vi "InitDrivebase.vi"   [LabVIEW 2023]
doc: "This VI initializes devices related directly to the drive subsystem."
uses:
  <vilib>/Rock Robotics/WPI/Solenoid/WPI_SolenoidChannel.ctl
  <vilib>/Rock Robotics/WPI/ThirdParty/Phoenix-LabVIEW/Motor Controller/Controls/CTRE_Phoenix_MotorControl_TalonFXInvertType.ctl
  <vilib>/Rock Robotics/WPI/ThirdParty/Phoenix-LabVIEW/Motor Controller/Controls/CTRE_Phoenix_MotorControl_SupplyCurrentLimitConfiguration.ctl
  <vilib>/Rock Robotics/WPI/ThirdParty/Phoenix-LabVIEW/Motor Controller/Controls/CTRE_Phoenix_MotorControl_NeutralMode.ctl
  <vilib>/Rock Robotics/WPI/ThirdParty/Phoenix-LabVIEW/Motor Controller/Controls/CTRE_Phoenix_MotorControl_FeedbackDevice_TalonFX.ctl
  <vilib>/Rock Robotics/WPI/ThirdParty/Phoenix-LabVIEW/Motor Controller/Controls/CTRE_Phoenix_MotorControl_StatusFrameEnhanced.ctl
  <vilib>/Rock Robotics/WPI/ThirdParty/Phoenix-LabVIEW/Motor Controller/Controls/CTRE_Phoenix_MotorControl_StatorCurrentLimitConfiguration.ctl
  <vilib>/Rock Robotics/WPI/Solenoid/WPI_SolenoidOpenDouble.vi
  GlobalDrivebase.vi
types:
  T1 = typedef "CTRE_Phoenix_MotorControl_StatorCurrentLimitConfiguration.ctl" = cluster{"Enable?":bool, "Current Limit":dbl, "Threshold Current":dbl, "Threshold Time":dbl}
  T2 = typedef "CTRE_Phoenix_MotorControl_StatusFrameEnhanced.ctl" = u16
  T3 = typedef "WPI_SolenoidChannel.ctl" = enum8{"Solenoid 0", "Solenoid 1", "Solenoid 2", "Solenoid 3", "Solenoid 4", "Solenoid 5", "Solenoid 6", "Solenoid 7", "Solenoid 8", "Solenoid 9", "Solenoid 10", "Solenoid 11", "Solenoid 12", "Solenoid 13", "Solenoid 14", "Solenoid 15", "Invalid"}
  T4 = typedef "CTRE_Phoenix_MotorControl_TalonFXInvertType.ctl" = enum16{"Counter-Clockwise", "Clockwise"}
  T5 = typedef "CTRE_Phoenix_MotorControl_FeedbackDevice_TalonFX.ctl" = i8
  T6 = typedef "CTRE_Phoenix_MotorControl_SupplyCurrentLimitConfiguration.ctl" = cluster{"Enable?":bool, "Current Limit":dbl, "Threshold Current":dbl, "Threshold Time":dbl}
  T7 = typedef "CTRE_Phoenix_MotorControl_NeutralMode.ctl" = enum8{"EEPROMSetting", "Override to Coast", "Override to Brake"}
  T8 = typedef "CTRE_PigeonIMU_DeviceRef.ctl" = cluster{"DeviceStatus":errorcluster, "Device Number":u8, "Type":T9, "Device ID":u32, "Handle":u64, "UsageFrame":u32, "Library Path":path}
  T9 = typedef "CTRE_PigeonIMU_ConnectionType.ctl" = u32
  T10 = typedef "WPI_MotorControlDeviceRef.ctl" = cluster{"DeviceStatus":errorcluster, "Type":T11, "PWM":cluster{"PWM Channel":T12, "DeadBand":T13}, "CAN":cluster{"Device Number":u8, "SetOutput VI Ref":variant, "GetOutput VI Ref":variant, "Enable VI Ref":variant, "Disable VI Ref":variant, "Data":variant}, "Invert":bool, "DIO PWM":cluster{"PWM \"Enable\" Channel":T12, "DIOChannel":T14, "PWM Rate":dbl}}
  T11 = typedef "WPI_MotorControlType.ctl" = enum16{"PWM", "CAN", "DIO PWM"}
  T12 = typedef "FPGA_DIOPWMChannel.ctl" = enum8{"PWM 0", "PWM 1", "PWM 2", "PWM 3", "PWM 4", "PWM 5", "PWM 6", "PWM 7", "PWM 8", "PWM 9", "PWM MXP 0", "PWM MXP 1", "PWM MXP 2", "PWM MXP 3", "PWM MXP 4", "PWM MXP 5", "PWM MXP 6", "PWM MXP 7", "PWM MXP 8", "PWM MXP 9", "Invalid"}
  T13 = typedef "WPI_PWMDeadband.ctl" = cluster{"Name":string, "maxPositivePwm":i32, "minPositivePwm":i32, "centerPwm":i32, "maxNegativePwm":i32, "minNegativePwm":i32, "angularRange":u16}
  T14 = typedef "FPGA_DIOChannel.ctl" = enum8{"DIO 0", "DIO 1", "DIO 2", "DIO 3", "DIO 4", "DIO 5", "DIO 6", "DIO 7", "DIO 8", "DIO 9", "DIO MXP 0", "DIO MXP 1", "DIO MXP 2", "DIO MXP 3", "DIO MXP 4", "DIO MXP 5", "DIO MXP 6", "DIO MXP 7", "DIO MXP 8", "DIO MXP 9", "DIO MXP 10", "DIO MXP 11", "DIO MXP 12", "DIO MXP 13", "DIO MXP 14", "DIO MXP 15", "SPI Port CS1", "SPI Port CS2", "SPI Port CS3", "SPI Port MISO", "SPI Port MOSI", "Invalid"}
  T15 = typedef "WPI_SolenoidDevRef.ctl" = cluster{"DevStatus":errorcluster, "Pneumatics Control Module":u8, "Forward Solenoid Channel":T3, "Reverse Solenoid Channel":T3}
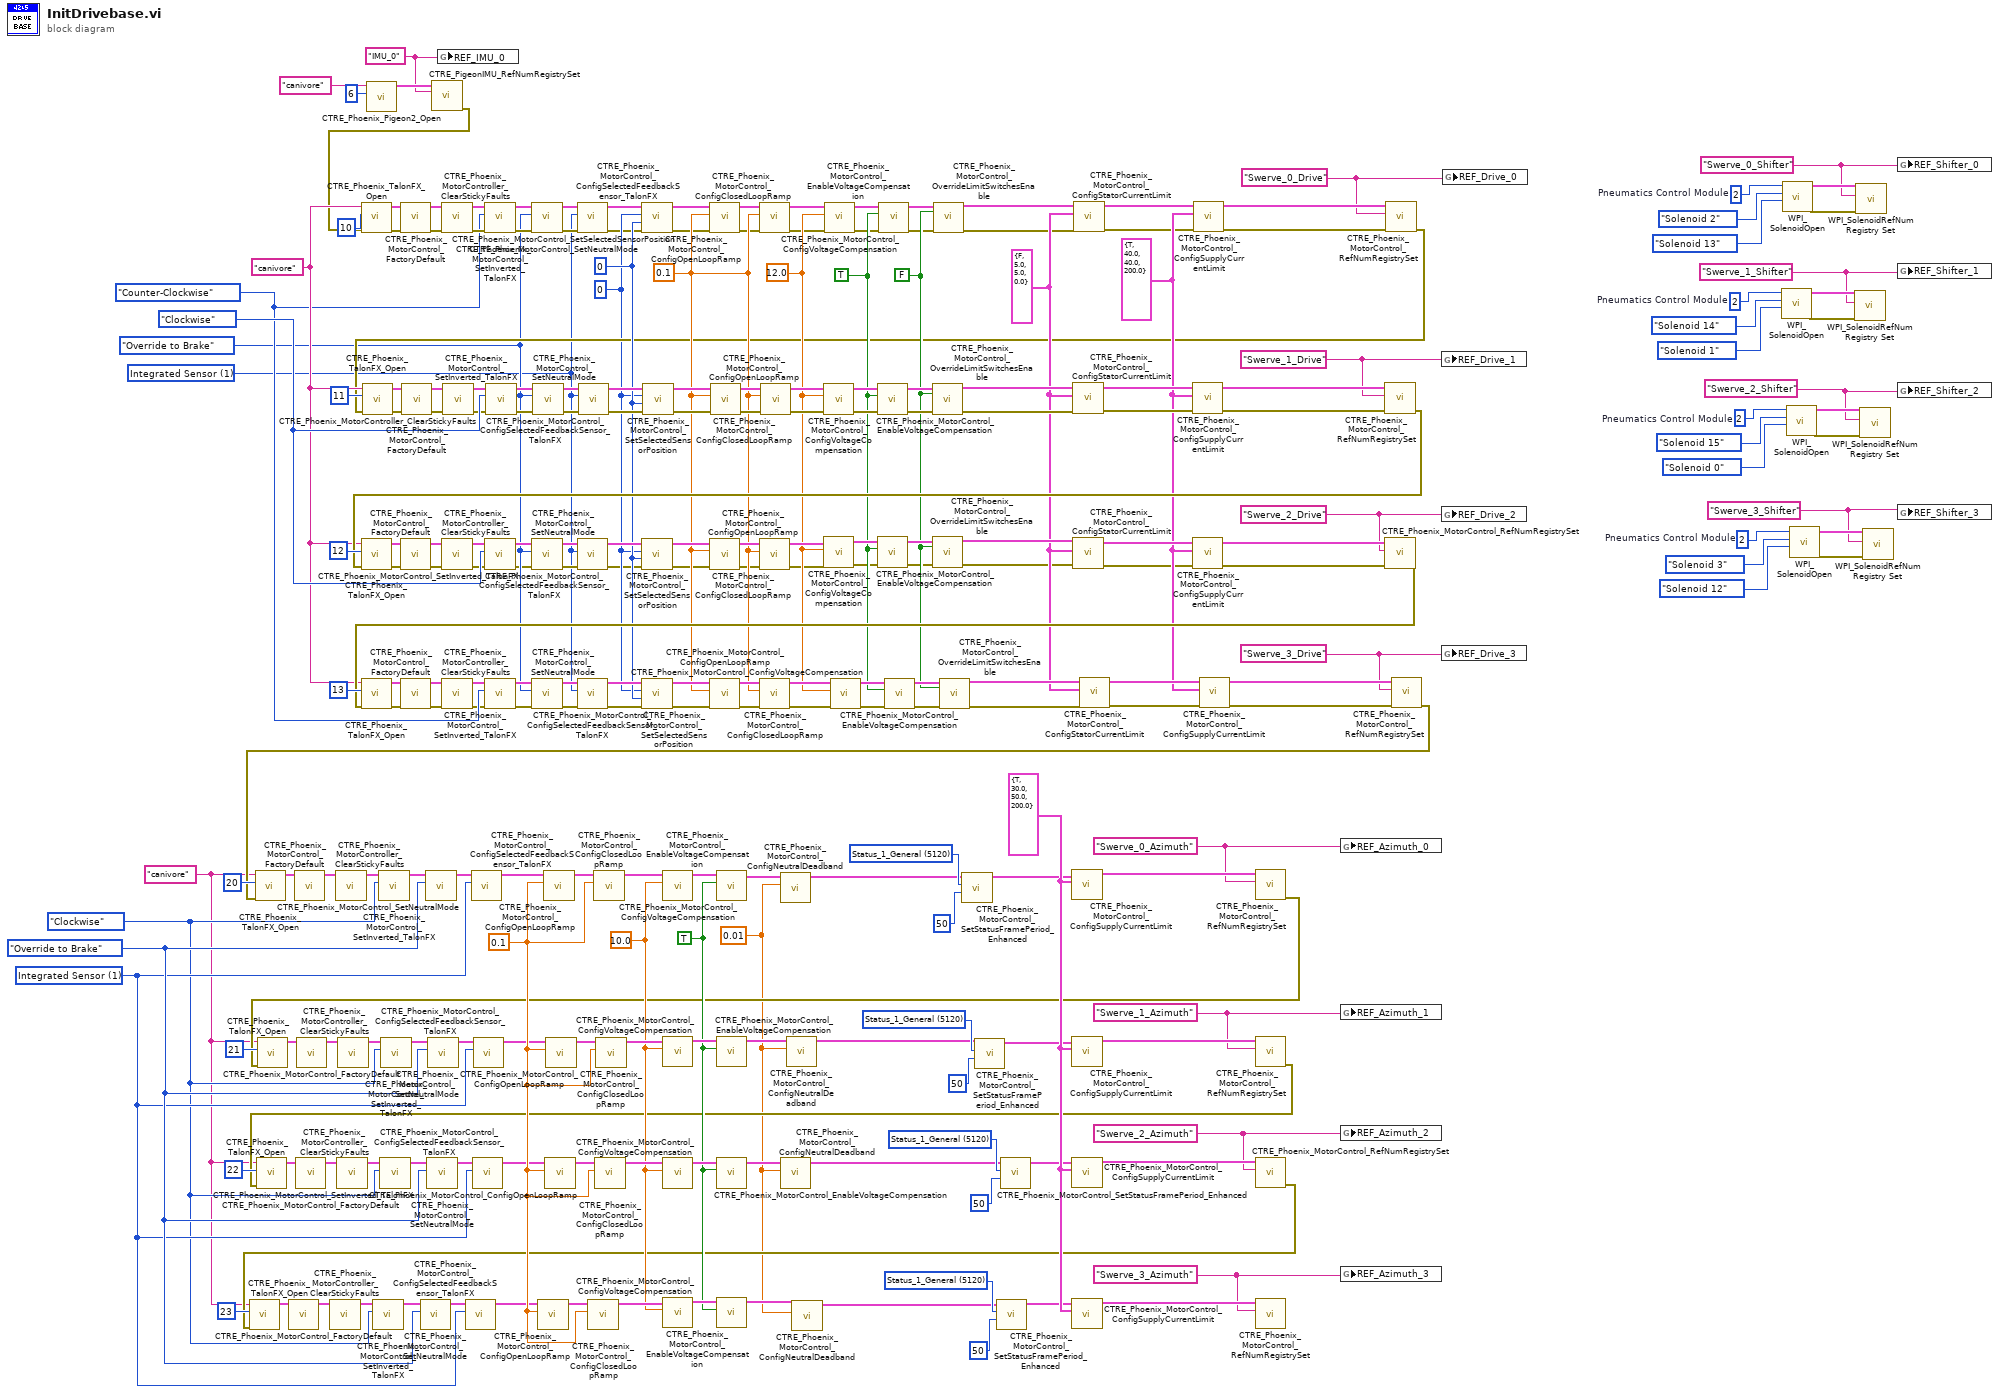
[diagram p0: block diagram]
diagram:
  w35 = "Swerve_0_Drive" ("refnum name")
  w64 = 0 ("New Sensor Position")
  w88 = "canivore" ("CAN Bus")
  w66 = "canivore" ("CAN Bus")
  w89 = "IMU_0" ("refnum name")
  w106 = 0.01 ("Percent Deadband")
  w73 = T1 {"Enable?"=FALSE, "Current Limit"=5.0, "Threshold Current"=5.0, "Threshold Time"=0.0} ("Stator Current Limit Configuration")
  w122 = T2 5120 items=["Status_1_General"=5120, "Status_2_Feedback0"=5184, "Status_3_Quadrature"=5248, "Status_4_AinTempVbat"=5312, "Status_6_Misc"=5440, "Status_7_CommStatus"=5504, "Status_8_PulseWidth"=5568, "Status_9_MotProfBuffer"=5632, "Status_10_MotionMagic"=5696, "Status_11_UartGadgeteer"=5760, "Status_12_Feedback1"=5824, "Status_13_Base_PIDF0"=5888, "Status_14_Turn_PIDF1"=5952, "Status_15_FirmwareApiStatus"=6016, "Status_Brushless_Current"=4672] ("Status Frame")
  w125 = T2 5120 items=["Status_1_General"=5120, "Status_2_Feedback0"=5184, "Status_3_Quadrature"=5248, "Status_4_AinTempVbat"=5312, "Status_6_Misc"=5440, "Status_7_CommStatus"=5504, "Status_8_PulseWidth"=5568, "Status_9_MotProfBuffer"=5632, "Status_10_MotionMagic"=5696, "Status_11_UartGadgeteer"=5760, "Status_12_Feedback1"=5824, "Status_13_Base_PIDF0"=5888, "Status_14_Turn_PIDF1"=5952, "Status_15_FirmwareApiStatus"=6016, "Status_Brushless_Current"=4672] ("Status Frame")
  w128 = T2 5120 items=["Status_1_General"=5120, "Status_2_Feedback0"=5184, "Status_3_Quadrature"=5248, "Status_4_AinTempVbat"=5312, "Status_6_Misc"=5440, "Status_7_CommStatus"=5504, "Status_8_PulseWidth"=5568, "Status_9_MotProfBuffer"=5632, "Status_10_MotionMagic"=5696, "Status_11_UartGadgeteer"=5760, "Status_12_Feedback1"=5824, "Status_13_Base_PIDF0"=5888, "Status_14_Turn_PIDF1"=5952, "Status_15_FirmwareApiStatus"=6016, "Status_Brushless_Current"=4672] ("Status Frame")
  w130 = T2 5120 items=["Status_1_General"=5120, "Status_2_Feedback0"=5184, "Status_3_Quadrature"=5248, "Status_4_AinTempVbat"=5312, "Status_6_Misc"=5440, "Status_7_CommStatus"=5504, "Status_8_PulseWidth"=5568, "Status_9_MotProfBuffer"=5632, "Status_10_MotionMagic"=5696, "Status_11_UartGadgeteer"=5760, "Status_12_Feedback1"=5824, "Status_13_Base_PIDF0"=5888, "Status_14_Turn_PIDF1"=5952, "Status_15_FirmwareApiStatus"=6016, "Status_Brushless_Current"=4672] ("Status Frame")
  w72 = FALSE ("Override Limit Switch Enable?")
  w100 = "Swerve_0_Shifter" ("refnum name")
  w148 = u8 2  # Pneumatics Control Module
  w99 = "Swerve_1_Shifter" ("refnum name")
  w153 = u8 2  # Pneumatics Control Module
  w98 = "Swerve_2_Shifter" ("refnum name")
  w158 = u8 2  # Pneumatics Control Module
  w32 = CTRE_Phoenix_MotorControl_TalonFXInvertType."Counter-Clockwise" ("Invert Type")
  w160 = TRUE ("Enable Voltage Compensation?")
  w161 = 10.0 ("Saturation Voltage")
  w71 = TRUE ("Enable Voltage Compensation?")
  w70 = 12.0 ("Saturation Voltage")
  w176 = T5 1 items=["Integrated Sensor"=1, "Sensor Sum (S0 + S1)"=9, "Sensor Difference (D0 - D1)"=10, "Remote Source 0"=11, "Remote Source 1"=12, "None"=14, "Software Emulated"=15] ("Talon FX Feedback Device")
  w179 = T6 {"Enable?"=TRUE, "Current Limit"=30.0, "Threshold Current"=50.0, "Threshold Time"=200.0} ("Supply Current Limit Configuration")
  w177 = 0.1 ("secondsFromNeutralToFull")
  w178 = CTRE_Phoenix_MotorControl_NeutralMode."Override to Brake" ("Motor Control Neutral Mode")
  w143 = CTRE_Phoenix_MotorControl_TalonFXInvertType."Clockwise" ("Invert Type")
  w93 = "Swerve_0_Azimuth" ("refnum name")
  w92 = "Swerve_1_Azimuth" ("refnum name")
  w91 = "Swerve_2_Azimuth" ("refnum name")
  w90 = "Swerve_3_Azimuth" ("refnum name")
  w1 = T5 1 items=["Integrated Sensor"=1, "Sensor Sum (S0 + S1)"=9, "Sensor Difference (D0 - D1)"=10, "Remote Source 0"=11, "Remote Source 1"=12, "None"=14, "Software Emulated"=15] ("Talon FX Feedback Device")
  w69 = T6 {"Enable?"=TRUE, "Current Limit"=40.0, "Threshold Current"=40.0, "Threshold Time"=200.0} ("Supply Current Limit Configuration")
  w68 = 0.1 ("secondsFromNeutralToFull")
  w67 = u32 0 ("pidLoopIdx")
  w31 = CTRE_Phoenix_MotorControl_NeutralMode."Override to Brake" ("Motor Control Neutral Mode")
  w159 = CTRE_Phoenix_MotorControl_TalonFXInvertType."Clockwise" ("Invert Type")
  w96 = "Swerve_1_Drive" ("refnum name")
  w95 = "Swerve_2_Drive" ("refnum name")
  w94 = "Swerve_3_Drive" ("refnum name")
  w97 = "Swerve_3_Shifter" ("refnum name")
  w246 = u8 2  # Pneumatics Control Module
  n1 = call <vilib>:"CTRE_Phoenix_Pigeon2_Open.vi"("Device Number"=u8 6, "canbus"="canivore") -> ("PigeonIMUDevRef"=w104:T8)  [unwired: 8 in, 1 out]
  n2 = call <vilib>:"CTRE_PigeonIMU_RefNumRegistrySet.vi"("refnum name"=w89, "PigeonIMUDevRef"=w104) -> ("error out"=w33:errorcluster)  [unwired: 8 in, 1 out]
  n3 = call <vilib>:"CTRE_Phoenix_TalonFX_Open.vi"("error in"=w33, "Device Number"=u8 10 ("Drive 4L"), "CAN Bus"=w66) -> ("error out"=w50:errorcluster, "PhoenixMotorControlDevRef"=w39:T10)  [unwired: 7 in]
  n4 = call <vilib>:"CTRE_Phoenix_MotorControl_FactoryDefault.vi"("error in"=w50, "PhoenixMotorControlDevRef"=w39) -> ("error out"=w51:errorcluster, "PhoenixMotorControlDevRef"=w41:T10)  [unwired: 8 in]
  n5 = global write "GlobalDrivebase.vi" "REF_IMU_0"(w89) -> ()
  n6 = call <vilib>:"CTRE_Phoenix_MotorController_ClearStickyFaults.vi"("error in"=w51, "PhoenixMotorControlDevRef"=w41) -> ("error out"=w52:errorcluster, "PhoenixMotorControlDevRef"=w42:T10)  [unwired: 8 in]
  n7 = call <vilib>:"CTRE_Phoenix_MotorControl_SetInverted_TalonFX.vi"("error in (no error)"=w52, "Invert Type"=w32, "PhoenixMotorControlDevRef"=w42) -> ("error out"=w53:errorcluster, "PhoenixMotorControlDevRef"=w36:T10)  [unwired: 7 in]
  n8 = call <vilib>:"CTRE_Phoenix_MotorControl_SetNeutralMode.vi"("error in (no error)"=w53, "Motor Control Neutral Mode"=w31, "PhoenixMotorControlDevRef"=w36) -> ("error out"=w54:errorcluster, "PhoenixMotorControlDevRef"=w43:T10)  [unwired: 7 in]
  n9 = call <vilib>:"CTRE_Phoenix_MotorControl_ConfigSelectedFeedbackSensor_TalonFX.vi"("error in (no error)"=w54, "Talon FX Feedback Device"=w1, "PhoenixMotorControlDevRef"=w43) -> ("error out"=w55:errorcluster, "PhoenixMotorControlDevRef"=w44:T10)  [unwired: 7 in]
  n10 = call <vilib>:"CTRE_Phoenix_MotorControl_SetSelectedSensorPosition.vi"("error in (no error)"=w55, "pidLoopIdx"=w67, "New Sensor Position"=w64, "PhoenixMotorControlDevRef"=w44) -> ("error out"=w56:errorcluster, "PhoenixMotorControlDevRef"=w37:T10)  [unwired: 6 in]
  n11 = call <vilib>:"CTRE_Phoenix_MotorControl_ConfigOpenLoopRamp.vi"("error in (no error)"=w56, "secondsFromNeutralToFull"=w68, "PhoenixMotorControlDevRef"=w37) -> ("error out"=w57:errorcluster, "PhoenixMotorControlDevRef"=w40:T10)  [unwired: 7 in]
  n12 = call <vilib>:"CTRE_Phoenix_MotorControl_ConfigClosedLoopRamp.vi"("error in (no error)"=w57, "secondsFromNeutralToFull"=w68, "PhoenixMotorControlDevRef"=w40) -> ("error out"=w58:errorcluster, "PhoenixMotorControlDevRef"=w46:T10)  [unwired: 7 in]
  n13 = call <vilib>:"CTRE_Phoenix_MotorControl_ConfigVoltageCompensation.vi"("error in (no error)"=w58, "Saturation Voltage"=w70, "PhoenixMotorControlDevRef"=w46) -> ("error out"=w59:errorcluster, "PhoenixMotorControlDevRef"=w45:T10)  [unwired: 7 in]
  n14 = call <vilib>:"CTRE_Phoenix_MotorControl_EnableVoltageCompensation.vi"("error in (no error)"=w59, "Enable Voltage Compensation?"=w71, "PhoenixMotorControlDevRef"=w45) -> ("error out"=w60:errorcluster, "PhoenixMotorControlDevRef"=w47:T10)  [unwired: 7 in]
  n15 = call <vilib>:"CTRE_Phoenix_MotorControl_OverrideLimitSwitchesEnable.vi"("PhoenixMotorControlDevRef"=w47, "Override Limit Switch Enable?"=w72, "error in (no error)"=w60) -> ("PhoenixMotorControlDevRef"=w49:T10, "error out"=w61:errorcluster)  [unwired: 11 in]
  n16 = call <vilib>:"CTRE_Phoenix_MotorControl_ConfigStatorCurrentLimit.vi"("error in (no error)"=w61, "Stator Current Limit Configuration"=w73, "PhoenixMotorControlDevRef"=w49) -> ("error out"=w62:errorcluster, "PhoenixMotorControlDevRef"=w48:T10)  [unwired: 7 in]
  n17 = call <vilib>:"CTRE_Phoenix_MotorControl_ConfigSupplyCurrentLimit.vi"("error in (no error)"=w62, "Supply Current Limit Configuration"=w69, "PhoenixMotorControlDevRef"=w48) -> ("error out"=w63:errorcluster, "PhoenixMotorControlDevRef"=w38:T10)  [unwired: 7 in]
  n18 = global write "GlobalDrivebase.vi" "REF_Azimuth_0"(w93) -> ()
  n19 = global write "GlobalDrivebase.vi" "REF_Azimuth_1"(w92) -> ()
  n20 = global write "GlobalDrivebase.vi" "REF_Azimuth_2"(w91) -> ()
  n21 = global write "GlobalDrivebase.vi" "REF_Azimuth_3"(w90) -> ()
  n22 = call <vilib>:"CTRE_Phoenix_MotorControl_RefNumRegistrySet.vi"("error in (no error)"=w63, "refnum name"=w35, "PhoenixMotorControlDevRef"=w38) -> ("error out"=w65:errorcluster)  [unwired: 7 in, 1 out]
  n23 = call <vilib>:"CTRE_Phoenix_TalonFX_Open.vi"("error in"=w65, "Device Number"=u8 11 ("Drive 4L"), "CAN Bus"=w66) -> ("error out"=w86:errorcluster, "PhoenixMotorControlDevRef"=w217:T10)  [unwired: 7 in]
  n24 = call <vilib>:"CTRE_Phoenix_MotorControl_FactoryDefault.vi"("error in"=w86, "PhoenixMotorControlDevRef"=w217) -> ("error out"=w85:errorcluster, "PhoenixMotorControlDevRef"=w215:T10)  [unwired: 8 in]
  n25 = call <vilib>:"CTRE_Phoenix_MotorController_ClearStickyFaults.vi"("error in"=w85, "PhoenixMotorControlDevRef"=w215) -> ("error out"=w84:errorcluster, "PhoenixMotorControlDevRef"=w214:T10)  [unwired: 8 in]
  n26 = call <vilib>:"CTRE_Phoenix_MotorControl_SetInverted_TalonFX.vi"("error in (no error)"=w84, "Invert Type"=w159, "PhoenixMotorControlDevRef"=w214) -> ("error out"=w83:errorcluster, "PhoenixMotorControlDevRef"=w221:T10)  [unwired: 7 in]
  n27 = call <vilib>:"CTRE_Phoenix_MotorControl_SetNeutralMode.vi"("error in (no error)"=w83, "Motor Control Neutral Mode"=w31, "PhoenixMotorControlDevRef"=w221) -> ("error out"=w82:errorcluster, "PhoenixMotorControlDevRef"=w213:T10)  [unwired: 7 in]
  n28 = call <vilib>:"CTRE_Phoenix_MotorControl_ConfigSelectedFeedbackSensor_TalonFX.vi"("error in (no error)"=w82, "Talon FX Feedback Device"=w1, "PhoenixMotorControlDevRef"=w213) -> ("error out"=w81:errorcluster, "PhoenixMotorControlDevRef"=w212:T10)  [unwired: 7 in]
  n29 = call <vilib>:"CTRE_Phoenix_MotorControl_SetSelectedSensorPosition.vi"("error in (no error)"=w81, "pidLoopIdx"=w67, "New Sensor Position"=w64, "PhoenixMotorControlDevRef"=w212) -> ("error out"=w80:errorcluster, "PhoenixMotorControlDevRef"=w220:T10)  [unwired: 6 in]
  n30 = call <vilib>:"CTRE_Phoenix_MotorControl_ConfigOpenLoopRamp.vi"("error in (no error)"=w80, "secondsFromNeutralToFull"=w68, "PhoenixMotorControlDevRef"=w220) -> ("error out"=w79:errorcluster, "PhoenixMotorControlDevRef"=w216:T10)  [unwired: 7 in]
  n31 = call <vilib>:"CTRE_Phoenix_MotorControl_ConfigClosedLoopRamp.vi"("error in (no error)"=w79, "secondsFromNeutralToFull"=w68, "PhoenixMotorControlDevRef"=w216) -> ("error out"=w78:errorcluster, "PhoenixMotorControlDevRef"=w168:T10)  [unwired: 7 in]
  n32 = call <vilib>:"CTRE_Phoenix_MotorControl_ConfigVoltageCompensation.vi"("error in (no error)"=w78, "Saturation Voltage"=w70, "PhoenixMotorControlDevRef"=w168) -> ("error out"=w77:errorcluster, "PhoenixMotorControlDevRef"=w175:T10)  [unwired: 7 in]
  n33 = call <vilib>:"CTRE_Phoenix_MotorControl_EnableVoltageCompensation.vi"("error in (no error)"=w77, "Enable Voltage Compensation?"=w71, "PhoenixMotorControlDevRef"=w175) -> ("error out"=w76:errorcluster, "PhoenixMotorControlDevRef"=w142:T10)  [unwired: 7 in]
  n34 = call <vilib>:"CTRE_Phoenix_MotorControl_OverrideLimitSwitchesEnable.vi"("PhoenixMotorControlDevRef"=w142, "Override Limit Switch Enable?"=w72, "error in (no error)"=w76) -> ("PhoenixMotorControlDevRef"=w117:T10, "error out"=w75:errorcluster)  [unwired: 11 in]
  n35 = call <vilib>:"CTRE_Phoenix_MotorControl_ConfigStatorCurrentLimit.vi"("error in (no error)"=w75, "Stator Current Limit Configuration"=w73, "PhoenixMotorControlDevRef"=w117) -> ("error out"=w74:errorcluster, "PhoenixMotorControlDevRef"=w120:T10)  [unwired: 7 in]
  n36 = call <vilib>:"CTRE_Phoenix_MotorControl_ConfigSupplyCurrentLimit.vi"("error in (no error)"=w74, "Supply Current Limit Configuration"=w69, "PhoenixMotorControlDevRef"=w120) -> ("error out"=w30:errorcluster, "PhoenixMotorControlDevRef"=w219:T10)  [unwired: 7 in]
  n37 = call <vilib>:"CTRE_Phoenix_MotorControl_RefNumRegistrySet.vi"("error in (no error)"=w30, "refnum name"=w96, "PhoenixMotorControlDevRef"=w219) -> ("error out"=w103:errorcluster)  [unwired: 7 in, 1 out]
  n38 = call <vilib>:"CTRE_Phoenix_TalonFX_Open.vi"("error in"=w103, "Device Number"=u8 12 ("Drive 4L"), "CAN Bus"=w66) -> ("error out"=w29:errorcluster, "PhoenixMotorControlDevRef"=w227:T10)  [unwired: 7 in]
  n39 = call <vilib>:"CTRE_Phoenix_MotorControl_FactoryDefault.vi"("error in"=w29, "PhoenixMotorControlDevRef"=w227) -> ("error out"=w28:errorcluster, "PhoenixMotorControlDevRef"=w225:T10)  [unwired: 8 in]
  n40 = call <vilib>:"CTRE_Phoenix_MotorController_ClearStickyFaults.vi"("error in"=w28, "PhoenixMotorControlDevRef"=w225) -> ("error out"=w27:errorcluster, "PhoenixMotorControlDevRef"=w224:T10)  [unwired: 8 in]
  n41 = call <vilib>:"CTRE_Phoenix_MotorControl_SetInverted_TalonFX.vi"("error in (no error)"=w27, "Invert Type"=w159, "PhoenixMotorControlDevRef"=w224) -> ("error out"=w26:errorcluster, "PhoenixMotorControlDevRef"=w231:T10)  [unwired: 7 in]
  n42 = call <vilib>:"CTRE_Phoenix_MotorControl_SetNeutralMode.vi"("error in (no error)"=w26, "Motor Control Neutral Mode"=w31, "PhoenixMotorControlDevRef"=w231) -> ("error out"=w25:errorcluster, "PhoenixMotorControlDevRef"=w223:T10)  [unwired: 7 in]
  n43 = call <vilib>:"CTRE_Phoenix_MotorControl_ConfigSelectedFeedbackSensor_TalonFX.vi"("error in (no error)"=w25, "Talon FX Feedback Device"=w1, "PhoenixMotorControlDevRef"=w223) -> ("error out"=w24:errorcluster, "PhoenixMotorControlDevRef"=w222:T10)  [unwired: 7 in]
  n44 = call <vilib>:"CTRE_Phoenix_MotorControl_SetSelectedSensorPosition.vi"("error in (no error)"=w24, "pidLoopIdx"=w67, "New Sensor Position"=w64, "PhoenixMotorControlDevRef"=w222) -> ("error out"=w23:errorcluster, "PhoenixMotorControlDevRef"=w230:T10)  [unwired: 6 in]
  n45 = call <vilib>:"CTRE_Phoenix_MotorControl_ConfigOpenLoopRamp.vi"("error in (no error)"=w23, "secondsFromNeutralToFull"=w68, "PhoenixMotorControlDevRef"=w230) -> ("error out"=w22:errorcluster, "PhoenixMotorControlDevRef"=w226:T10)  [unwired: 7 in]
  n46 = call <vilib>:"CTRE_Phoenix_MotorControl_ConfigClosedLoopRamp.vi"("error in (no error)"=w22, "secondsFromNeutralToFull"=w68, "PhoenixMotorControlDevRef"=w226) -> ("error out"=w21:errorcluster, "PhoenixMotorControlDevRef"=w167:T10)  [unwired: 7 in]
  n47 = call <vilib>:"CTRE_Phoenix_MotorControl_ConfigVoltageCompensation.vi"("error in (no error)"=w21, "Saturation Voltage"=w70, "PhoenixMotorControlDevRef"=w167) -> ("error out"=w20:errorcluster, "PhoenixMotorControlDevRef"=w174:T10)  [unwired: 7 in]
  n48 = call <vilib>:"CTRE_Phoenix_MotorControl_EnableVoltageCompensation.vi"("error in (no error)"=w20, "Enable Voltage Compensation?"=w71, "PhoenixMotorControlDevRef"=w174) -> ("error out"=w19:errorcluster, "PhoenixMotorControlDevRef"=w141:T10)  [unwired: 7 in]
  n49 = call <vilib>:"CTRE_Phoenix_MotorControl_OverrideLimitSwitchesEnable.vi"("PhoenixMotorControlDevRef"=w141, "Override Limit Switch Enable?"=w72, "error in (no error)"=w19) -> ("PhoenixMotorControlDevRef"=w116:T10, "error out"=w18:errorcluster)  [unwired: 11 in]
  n50 = call <vilib>:"CTRE_Phoenix_MotorControl_ConfigStatorCurrentLimit.vi"("error in (no error)"=w18, "Stator Current Limit Configuration"=w73, "PhoenixMotorControlDevRef"=w116) -> ("error out"=w17:errorcluster, "PhoenixMotorControlDevRef"=w119:T10)  [unwired: 7 in]
  n51 = call <vilib>:"CTRE_Phoenix_MotorControl_ConfigSupplyCurrentLimit.vi"("error in (no error)"=w17, "Supply Current Limit Configuration"=w69, "PhoenixMotorControlDevRef"=w119) -> ("error out"=w16:errorcluster, "PhoenixMotorControlDevRef"=w229:T10)  [unwired: 7 in]
  n52 = call <vilib>:"CTRE_Phoenix_MotorControl_RefNumRegistrySet.vi"("error in (no error)"=w16, "refnum name"=w95, "PhoenixMotorControlDevRef"=w229) -> ("error out"=w102:errorcluster)  [unwired: 7 in, 1 out]
  n53 = call <vilib>:"CTRE_Phoenix_TalonFX_Open.vi"("error in"=w102, "Device Number"=u8 13 ("Drive 4L"), "CAN Bus"=w66) -> ("error out"=w15:errorcluster, "PhoenixMotorControlDevRef"=w237:T10)  [unwired: 7 in]
  n54 = call <vilib>:"CTRE_Phoenix_MotorControl_FactoryDefault.vi"("error in"=w15, "PhoenixMotorControlDevRef"=w237) -> ("error out"=w14:errorcluster, "PhoenixMotorControlDevRef"=w235:T10)  [unwired: 8 in]
  n55 = call <vilib>:"CTRE_Phoenix_MotorController_ClearStickyFaults.vi"("error in"=w14, "PhoenixMotorControlDevRef"=w235) -> ("error out"=w13:errorcluster, "PhoenixMotorControlDevRef"=w234:T10)  [unwired: 8 in]
  n56 = call <vilib>:"CTRE_Phoenix_MotorControl_SetInverted_TalonFX.vi"("error in (no error)"=w13, "Invert Type"=w32, "PhoenixMotorControlDevRef"=w234) -> ("error out"=w12:errorcluster, "PhoenixMotorControlDevRef"=w241:T10)  [unwired: 7 in]
  n57 = call <vilib>:"CTRE_Phoenix_MotorControl_SetNeutralMode.vi"("error in (no error)"=w12, "Motor Control Neutral Mode"=w31, "PhoenixMotorControlDevRef"=w241) -> ("error out"=w11:errorcluster, "PhoenixMotorControlDevRef"=w233:T10)  [unwired: 7 in]
  n58 = call <vilib>:"CTRE_Phoenix_MotorControl_ConfigSelectedFeedbackSensor_TalonFX.vi"("error in (no error)"=w11, "Talon FX Feedback Device"=w1, "PhoenixMotorControlDevRef"=w233) -> ("error out"=w10:errorcluster, "PhoenixMotorControlDevRef"=w232:T10)  [unwired: 7 in]
  n59 = call <vilib>:"CTRE_Phoenix_MotorControl_SetSelectedSensorPosition.vi"("error in (no error)"=w10, "pidLoopIdx"=w67, "New Sensor Position"=w64, "PhoenixMotorControlDevRef"=w232) -> ("error out"=w9:errorcluster, "PhoenixMotorControlDevRef"=w240:T10)  [unwired: 6 in]
  n60 = call <vilib>:"CTRE_Phoenix_MotorControl_ConfigOpenLoopRamp.vi"("error in (no error)"=w9, "secondsFromNeutralToFull"=w68, "PhoenixMotorControlDevRef"=w240) -> ("error out"=w8:errorcluster, "PhoenixMotorControlDevRef"=w236:T10)  [unwired: 7 in]
  n61 = call <vilib>:"CTRE_Phoenix_MotorControl_ConfigClosedLoopRamp.vi"("error in (no error)"=w8, "secondsFromNeutralToFull"=w68, "PhoenixMotorControlDevRef"=w236) -> ("error out"=w7:errorcluster, "PhoenixMotorControlDevRef"=w166:T10)  [unwired: 7 in]
  n62 = call <vilib>:"CTRE_Phoenix_MotorControl_ConfigVoltageCompensation.vi"("error in (no error)"=w7, "Saturation Voltage"=w70, "PhoenixMotorControlDevRef"=w166) -> ("error out"=w6:errorcluster, "PhoenixMotorControlDevRef"=w173:T10)  [unwired: 7 in]
  n63 = call <vilib>:"CTRE_Phoenix_MotorControl_EnableVoltageCompensation.vi"("error in (no error)"=w6, "Enable Voltage Compensation?"=w71, "PhoenixMotorControlDevRef"=w173) -> ("error out"=w5:errorcluster, "PhoenixMotorControlDevRef"=w140:T10)  [unwired: 7 in]
  n64 = call <vilib>:"CTRE_Phoenix_MotorControl_OverrideLimitSwitchesEnable.vi"("PhoenixMotorControlDevRef"=w140, "Override Limit Switch Enable?"=w72, "error in (no error)"=w5) -> ("PhoenixMotorControlDevRef"=w115:T10, "error out"=w4:errorcluster)  [unwired: 11 in]
  n65 = call <vilib>:"CTRE_Phoenix_MotorControl_ConfigStatorCurrentLimit.vi"("error in (no error)"=w4, "Stator Current Limit Configuration"=w73, "PhoenixMotorControlDevRef"=w115) -> ("error out"=w3:errorcluster, "PhoenixMotorControlDevRef"=w118:T10)  [unwired: 7 in]
  n66 = call <vilib>:"CTRE_Phoenix_MotorControl_ConfigSupplyCurrentLimit.vi"("error in (no error)"=w3, "Supply Current Limit Configuration"=w69, "PhoenixMotorControlDevRef"=w118) -> ("error out"=w2:errorcluster, "PhoenixMotorControlDevRef"=w239:T10)  [unwired: 7 in]
  n67 = call <vilib>:"CTRE_Phoenix_MotorControl_RefNumRegistrySet.vi"("error in (no error)"=w2, "refnum name"=w94, "PhoenixMotorControlDevRef"=w239) -> ("error out"=w101:errorcluster)  [unwired: 7 in, 1 out]
  n68 = call <vilib>:"CTRE_Phoenix_TalonFX_Open.vi"("error in"=w101, "Device Number"=u8 20 ("Drive 4L"), "CAN Bus"=w88) -> ("PhoenixMotorControlDevRef"=w184:T10)  [unwired: 7 in, 1 out]
  n69 = call <vilib>:"CTRE_Phoenix_MotorControl_FactoryDefault.vi"("PhoenixMotorControlDevRef"=w184) -> ("PhoenixMotorControlDevRef"=w182:T10)  [unwired: 9 in, 1 out]
  n70 = call <vilib>:"CTRE_Phoenix_MotorController_ClearStickyFaults.vi"("PhoenixMotorControlDevRef"=w182) -> ("PhoenixMotorControlDevRef"=w181:T10)  [unwired: 9 in, 1 out]
  n71 = call <vilib>:"CTRE_Phoenix_MotorControl_SetInverted_TalonFX.vi"("Invert Type"=w143, "PhoenixMotorControlDevRef"=w181) -> ("PhoenixMotorControlDevRef"=w187:T10)  [unwired: 8 in, 1 out]
  n72 = call <vilib>:"CTRE_Phoenix_MotorControl_SetNeutralMode.vi"("Motor Control Neutral Mode"=w178, "PhoenixMotorControlDevRef"=w187) -> ("PhoenixMotorControlDevRef"=w180:T10)  [unwired: 8 in, 1 out]
  n73 = call <vilib>:"CTRE_Phoenix_MotorControl_ConfigSelectedFeedbackSensor_TalonFX.vi"("Talon FX Feedback Device"=w176, "PhoenixMotorControlDevRef"=w180) -> ("PhoenixMotorControlDevRef"=w136:T10)  [unwired: 8 in, 1 out]
  n74 = call <vilib>:"CTRE_Phoenix_MotorControl_ConfigOpenLoopRamp.vi"("secondsFromNeutralToFull"=w177, "PhoenixMotorControlDevRef"=w136) -> ("PhoenixMotorControlDevRef"=w183:T10)  [unwired: 8 in, 1 out]
  n75 = call <vilib>:"CTRE_Phoenix_MotorControl_ConfigClosedLoopRamp.vi"("secondsFromNeutralToFull"=w177, "PhoenixMotorControlDevRef"=w183) -> ("PhoenixMotorControlDevRef"=w165:T10)  [unwired: 8 in, 1 out]
  n76 = call <vilib>:"CTRE_Phoenix_MotorControl_ConfigVoltageCompensation.vi"("Saturation Voltage"=w161, "PhoenixMotorControlDevRef"=w165) -> ("PhoenixMotorControlDevRef"=w172:T10)  [unwired: 8 in, 1 out]
  n77 = call <vilib>:"CTRE_Phoenix_MotorControl_EnableVoltageCompensation.vi"("Enable Voltage Compensation?"=w160, "PhoenixMotorControlDevRef"=w172) -> ("PhoenixMotorControlDevRef"=w114:T10)  [unwired: 8 in, 1 out]
  n78 = call <vilib>:"CTRE_Phoenix_MotorControl_ConfigNeutralDeadband.vi"("Percent Deadband"=w106, "PhoenixMotorControlDevRef"=w114) -> ("PhoenixMotorControlDevRef"=w113:T10)  [unwired: 8 in, 1 out]
  n79 = call <vilib>:"CTRE_Phoenix_MotorControl_SetStatusFramePeriod_Enhanced.vi"("periodMs"=50, "Status Frame"=w130, "PhoenixMotorControlDevRef"=w113) -> ("PhoenixMotorControlDevRef"=w131:T10)  [unwired: 7 in, 1 out]
  n80 = call <vilib>:"CTRE_Phoenix_MotorControl_ConfigSupplyCurrentLimit.vi"("Supply Current Limit Configuration"=w179, "PhoenixMotorControlDevRef"=w131) -> ("PhoenixMotorControlDevRef"=w186:T10)  [unwired: 8 in, 1 out]
  n81 = call <vilib>:"CTRE_Phoenix_MotorControl_RefNumRegistrySet.vi"("refnum name"=w93, "PhoenixMotorControlDevRef"=w186) -> ("error out"=w135:errorcluster)  [unwired: 8 in, 1 out]
  n82 = call <vilib>:"CTRE_Phoenix_TalonFX_Open.vi"("error in"=w135, "Device Number"=u8 21 ("Drive 4L"), "CAN Bus"=w88) -> ("PhoenixMotorControlDevRef"=w192:T10)  [unwired: 7 in, 1 out]
  n83 = call <vilib>:"CTRE_Phoenix_MotorControl_FactoryDefault.vi"("PhoenixMotorControlDevRef"=w192) -> ("PhoenixMotorControlDevRef"=w190:T10)  [unwired: 9 in, 1 out]
  n84 = call <vilib>:"CTRE_Phoenix_MotorController_ClearStickyFaults.vi"("PhoenixMotorControlDevRef"=w190) -> ("PhoenixMotorControlDevRef"=w189:T10)  [unwired: 9 in, 1 out]
  n85 = call <vilib>:"CTRE_Phoenix_MotorControl_SetInverted_TalonFX.vi"("Invert Type"=w143, "PhoenixMotorControlDevRef"=w189) -> ("PhoenixMotorControlDevRef"=w195:T10)  [unwired: 8 in, 1 out]
  n86 = call <vilib>:"CTRE_Phoenix_MotorControl_SetNeutralMode.vi"("Motor Control Neutral Mode"=w178, "PhoenixMotorControlDevRef"=w195) -> ("PhoenixMotorControlDevRef"=w188:T10)  [unwired: 8 in, 1 out]
  n87 = call <vilib>:"CTRE_Phoenix_MotorControl_ConfigSelectedFeedbackSensor_TalonFX.vi"("Talon FX Feedback Device"=w176, "PhoenixMotorControlDevRef"=w188) -> ("PhoenixMotorControlDevRef"=w137:T10)  [unwired: 8 in, 1 out]
  n88 = call <vilib>:"CTRE_Phoenix_MotorControl_ConfigOpenLoopRamp.vi"("secondsFromNeutralToFull"=w177, "PhoenixMotorControlDevRef"=w137) -> ("PhoenixMotorControlDevRef"=w191:T10)  [unwired: 8 in, 1 out]
  n89 = call <vilib>:"CTRE_Phoenix_MotorControl_ConfigClosedLoopRamp.vi"("secondsFromNeutralToFull"=w177, "PhoenixMotorControlDevRef"=w191) -> ("PhoenixMotorControlDevRef"=w164:T10)  [unwired: 8 in, 1 out]
  n90 = call <vilib>:"CTRE_Phoenix_MotorControl_ConfigVoltageCompensation.vi"("Saturation Voltage"=w161, "PhoenixMotorControlDevRef"=w164) -> ("PhoenixMotorControlDevRef"=w171:T10)  [unwired: 8 in, 1 out]
  n91 = call <vilib>:"CTRE_Phoenix_MotorControl_EnableVoltageCompensation.vi"("Enable Voltage Compensation?"=w160, "PhoenixMotorControlDevRef"=w171) -> ("PhoenixMotorControlDevRef"=w112:T10)  [unwired: 8 in, 1 out]
  n92 = call <vilib>:"CTRE_Phoenix_MotorControl_ConfigNeutralDeadband.vi"("Percent Deadband"=w106, "PhoenixMotorControlDevRef"=w112) -> ("PhoenixMotorControlDevRef"=w111:T10)  [unwired: 8 in, 1 out]
  n93 = call <vilib>:"CTRE_Phoenix_MotorControl_SetStatusFramePeriod_Enhanced.vi"("periodMs"=50, "Status Frame"=w128, "PhoenixMotorControlDevRef"=w111) -> ("PhoenixMotorControlDevRef"=w127:T10)  [unwired: 7 in, 1 out]
  n94 = call <vilib>:"CTRE_Phoenix_MotorControl_ConfigSupplyCurrentLimit.vi"("Supply Current Limit Configuration"=w179, "PhoenixMotorControlDevRef"=w127) -> ("PhoenixMotorControlDevRef"=w194:T10)  [unwired: 8 in, 1 out]
  n95 = call <vilib>:"CTRE_Phoenix_MotorControl_RefNumRegistrySet.vi"("refnum name"=w92, "PhoenixMotorControlDevRef"=w194) -> ("error out"=w134:errorcluster)  [unwired: 8 in, 1 out]
  n96 = call <vilib>:"CTRE_Phoenix_TalonFX_Open.vi"("error in"=w134, "Device Number"=u8 22 ("Drive 4L"), "CAN Bus"=w88) -> ("PhoenixMotorControlDevRef"=w200:T10)  [unwired: 7 in, 1 out]
  n97 = call <vilib>:"CTRE_Phoenix_MotorControl_FactoryDefault.vi"("PhoenixMotorControlDevRef"=w200) -> ("PhoenixMotorControlDevRef"=w198:T10)  [unwired: 9 in, 1 out]
  n98 = call <vilib>:"CTRE_Phoenix_MotorController_ClearStickyFaults.vi"("PhoenixMotorControlDevRef"=w198) -> ("PhoenixMotorControlDevRef"=w197:T10)  [unwired: 9 in, 1 out]
  n99 = call <vilib>:"CTRE_Phoenix_MotorControl_SetInverted_TalonFX.vi"("Invert Type"=w143, "PhoenixMotorControlDevRef"=w197) -> ("PhoenixMotorControlDevRef"=w203:T10)  [unwired: 8 in, 1 out]
  n100 = call <vilib>:"CTRE_Phoenix_MotorControl_SetNeutralMode.vi"("Motor Control Neutral Mode"=w178, "PhoenixMotorControlDevRef"=w203) -> ("PhoenixMotorControlDevRef"=w196:T10)  [unwired: 8 in, 1 out]
  n101 = call <vilib>:"CTRE_Phoenix_MotorControl_ConfigSelectedFeedbackSensor_TalonFX.vi"("Talon FX Feedback Device"=w176, "PhoenixMotorControlDevRef"=w196) -> ("PhoenixMotorControlDevRef"=w138:T10)  [unwired: 8 in, 1 out]
  n102 = call <vilib>:"CTRE_Phoenix_MotorControl_ConfigOpenLoopRamp.vi"("secondsFromNeutralToFull"=w177, "PhoenixMotorControlDevRef"=w138) -> ("PhoenixMotorControlDevRef"=w199:T10)  [unwired: 8 in, 1 out]
  n103 = call <vilib>:"CTRE_Phoenix_MotorControl_ConfigClosedLoopRamp.vi"("secondsFromNeutralToFull"=w177, "PhoenixMotorControlDevRef"=w199) -> ("PhoenixMotorControlDevRef"=w163:T10)  [unwired: 8 in, 1 out]
  n104 = call <vilib>:"CTRE_Phoenix_MotorControl_ConfigVoltageCompensation.vi"("Saturation Voltage"=w161, "PhoenixMotorControlDevRef"=w163) -> ("PhoenixMotorControlDevRef"=w170:T10)  [unwired: 8 in, 1 out]
  n105 = call <vilib>:"CTRE_Phoenix_MotorControl_EnableVoltageCompensation.vi"("Enable Voltage Compensation?"=w160, "PhoenixMotorControlDevRef"=w170) -> ("PhoenixMotorControlDevRef"=w110:T10)  [unwired: 8 in, 1 out]
  n106 = call <vilib>:"CTRE_Phoenix_MotorControl_ConfigNeutralDeadband.vi"("Percent Deadband"=w106, "PhoenixMotorControlDevRef"=w110) -> ("PhoenixMotorControlDevRef"=w109:T10)  [unwired: 8 in, 1 out]
  n107 = call <vilib>:"CTRE_Phoenix_MotorControl_SetStatusFramePeriod_Enhanced.vi"("periodMs"=50, "Status Frame"=w125, "PhoenixMotorControlDevRef"=w109) -> ("PhoenixMotorControlDevRef"=w124:T10)  [unwired: 7 in, 1 out]
  n108 = call <vilib>:"CTRE_Phoenix_MotorControl_ConfigSupplyCurrentLimit.vi"("Supply Current Limit Configuration"=w179, "PhoenixMotorControlDevRef"=w124) -> ("PhoenixMotorControlDevRef"=w202:T10)  [unwired: 8 in, 1 out]
  n109 = call <vilib>:"CTRE_Phoenix_MotorControl_RefNumRegistrySet.vi"("refnum name"=w91, "PhoenixMotorControlDevRef"=w202) -> ("error out"=w133:errorcluster)  [unwired: 8 in, 1 out]
  n110 = call <vilib>:"CTRE_Phoenix_TalonFX_Open.vi"("error in"=w133, "Device Number"=u8 23 ("Drive 4L"), "CAN Bus"=w88) -> ("PhoenixMotorControlDevRef"=w208:T10)  [unwired: 7 in, 1 out]
  n111 = call <vilib>:"CTRE_Phoenix_MotorControl_FactoryDefault.vi"("PhoenixMotorControlDevRef"=w208) -> ("PhoenixMotorControlDevRef"=w206:T10)  [unwired: 9 in, 1 out]
  n112 = call <vilib>:"CTRE_Phoenix_MotorController_ClearStickyFaults.vi"("PhoenixMotorControlDevRef"=w206) -> ("PhoenixMotorControlDevRef"=w205:T10)  [unwired: 9 in, 1 out]
  n113 = call <vilib>:"CTRE_Phoenix_MotorControl_SetInverted_TalonFX.vi"("Invert Type"=w143, "PhoenixMotorControlDevRef"=w205) -> ("PhoenixMotorControlDevRef"=w211:T10)  [unwired: 8 in, 1 out]
  n114 = call <vilib>:"CTRE_Phoenix_MotorControl_SetNeutralMode.vi"("Motor Control Neutral Mode"=w178, "PhoenixMotorControlDevRef"=w211) -> ("PhoenixMotorControlDevRef"=w204:T10)  [unwired: 8 in, 1 out]
  n115 = call <vilib>:"CTRE_Phoenix_MotorControl_ConfigSelectedFeedbackSensor_TalonFX.vi"("Talon FX Feedback Device"=w176, "PhoenixMotorControlDevRef"=w204) -> ("PhoenixMotorControlDevRef"=w139:T10)  [unwired: 8 in, 1 out]
  n116 = call <vilib>:"CTRE_Phoenix_MotorControl_ConfigOpenLoopRamp.vi"("secondsFromNeutralToFull"=w177, "PhoenixMotorControlDevRef"=w139) -> ("PhoenixMotorControlDevRef"=w207:T10)  [unwired: 8 in, 1 out]
  n117 = call <vilib>:"CTRE_Phoenix_MotorControl_ConfigClosedLoopRamp.vi"("secondsFromNeutralToFull"=w177, "PhoenixMotorControlDevRef"=w207) -> ("PhoenixMotorControlDevRef"=w162:T10)  [unwired: 8 in, 1 out]
  n118 = call <vilib>:"CTRE_Phoenix_MotorControl_ConfigVoltageCompensation.vi"("Saturation Voltage"=w161, "PhoenixMotorControlDevRef"=w162) -> ("PhoenixMotorControlDevRef"=w169:T10)  [unwired: 8 in, 1 out]
  n119 = call <vilib>:"CTRE_Phoenix_MotorControl_EnableVoltageCompensation.vi"("Enable Voltage Compensation?"=w160, "PhoenixMotorControlDevRef"=w169) -> ("PhoenixMotorControlDevRef"=w108:T10)  [unwired: 8 in, 1 out]
  n120 = call <vilib>:"CTRE_Phoenix_MotorControl_ConfigNeutralDeadband.vi"("Percent Deadband"=w106, "PhoenixMotorControlDevRef"=w108) -> ("PhoenixMotorControlDevRef"=w107:T10)  [unwired: 8 in, 1 out]
  n121 = call <vilib>:"CTRE_Phoenix_MotorControl_SetStatusFramePeriod_Enhanced.vi"("periodMs"=50, "Status Frame"=w122, "PhoenixMotorControlDevRef"=w107) -> ("PhoenixMotorControlDevRef"=w121:T10)  [unwired: 7 in, 1 out]
  n122 = call <vilib>:"CTRE_Phoenix_MotorControl_ConfigSupplyCurrentLimit.vi"("Supply Current Limit Configuration"=w179, "PhoenixMotorControlDevRef"=w121) -> ("PhoenixMotorControlDevRef"=w210:T10)  [unwired: 8 in, 1 out]
  n123 = call <vilib>:"CTRE_Phoenix_MotorControl_RefNumRegistrySet.vi"("refnum name"=w90, "PhoenixMotorControlDevRef"=w210) -> ()  [unwired: 8 in, 2 out]
  n124 = global write "GlobalDrivebase.vi" "REF_Drive_1"(w96) -> ()
  n125 = global write "GlobalDrivebase.vi" "REF_Drive_2"(w95) -> ()
  n126 = global write "GlobalDrivebase.vi" "REF_Drive_3"(w94) -> ()
  n127 = global write "GlobalDrivebase.vi" "REF_Drive_0"(w35) -> ()
  n128 = call-poly <vilib>:"WPI_SolenoidOpen.vi"("Reverse Solenoid Channel"=WPI_SolenoidChannel."Solenoid 1", "Forward Solenoid Channel"=WPI_SolenoidChannel."Solenoid 14", "Pneumatics Device (def)"=w153) -> ("error out"=w149:errorcluster, "SolenoidDevRef"=w150:T15)  [unwired: 7 in]
  n129 = call-poly <vilib>:"WPI_SolenoidOpen.vi"("Reverse Solenoid Channel"=WPI_SolenoidChannel."Solenoid 13", "Forward Solenoid Channel"=WPI_SolenoidChannel."Solenoid 2", "Pneumatics Device (def)"=w148) -> ("error out"=w144:errorcluster, "SolenoidDevRef"=w145:T15)  [unwired: 7 in]
  n130 = call-poly <vilib>:"WPI_SolenoidOpen.vi"("Reverse Solenoid Channel"=WPI_SolenoidChannel."Solenoid 0", "Forward Solenoid Channel"=WPI_SolenoidChannel."Solenoid 15", "Pneumatics Device (def)"=w158) -> ("error out"=w154:errorcluster, "SolenoidDevRef"=w155:T15)  [unwired: 7 in]
  n131 = call-poly <vilib>:"WPI_SolenoidOpen.vi"("Reverse Solenoid Channel"=WPI_SolenoidChannel."Solenoid 12", "Forward Solenoid Channel"=WPI_SolenoidChannel."Solenoid 3", "Pneumatics Device (def)"=w246) -> ("error out"=w242:errorcluster, "SolenoidDevRef"=w243:T15)  [unwired: 7 in]
  n132 = call <vilib>:"WPI_SolenoidRefNum Registry Set.vi"("error in (no error)"=w149, "refnum name"=w99, "SolenoidDevRef"=w150) -> ()  [unwired: 7 in, 2 out]
  n133 = call <vilib>:"WPI_SolenoidRefNum Registry Set.vi"("error in (no error)"=w144, "refnum name"=w100, "SolenoidDevRef"=w145) -> ()  [unwired: 7 in, 2 out]
  n134 = call <vilib>:"WPI_SolenoidRefNum Registry Set.vi"("error in (no error)"=w154, "refnum name"=w98, "SolenoidDevRef"=w155) -> ()  [unwired: 7 in, 2 out]
  n135 = call <vilib>:"WPI_SolenoidRefNum Registry Set.vi"("error in (no error)"=w242, "refnum name"=w97, "SolenoidDevRef"=w243) -> ()  [unwired: 7 in, 2 out]
  n136 = global write "GlobalDrivebase.vi" "REF_Shifter_0"(w100) -> ()
  n137 = global write "GlobalDrivebase.vi" "REF_Shifter_1"(w99) -> ()
  n138 = global write "GlobalDrivebase.vi" "REF_Shifter_2"(w98) -> ()
  n139 = global write "GlobalDrivebase.vi" "REF_Shifter_3"(w97) -> ()
